vi "Parse Info Section.vi"(8 "error in":errorcluster, 11 "EDS in":refnum<class "EDS.lvclass">) -> (0 "error out":errorcluster, 3 "EDS out":refnum<class "EDS.lvclass">)   [LabVIEW 2024, in "EDS.lvlib" / "EDS.lvclass"]
uses:
  EDS.lvclass
  EDS.lvclass/EDS.ctl
  Device Info/Device Info.lvclass
  File Info/File Info.lvclass
  Info Section/Info Section.lvclass
  D:/git/EDS-File-Viewer/Core/Info Section/Info Section.lvclass
  D:/git/EDS-File-Viewer/Core/Device Info/Device Info.lvclass
  D:/git/EDS-File-Viewer/Core/File Info/File Info.lvclass
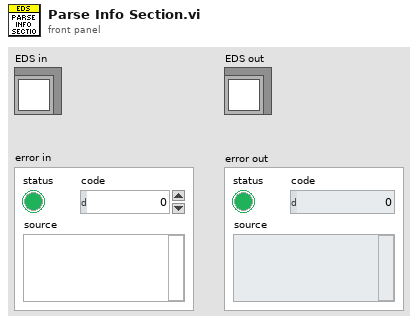
[diagram p1: front panel]
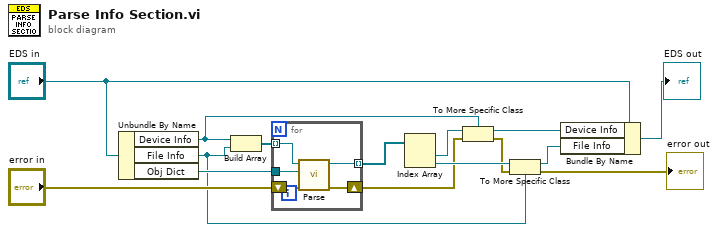
[diagram p0: block diagram]
diagram:
  n1 = Unbundle By Name("EDS in") -> ("Device Info"=w4:refnum<class "Device Info.lvclass">, "File Info"=w7:refnum<class "File Info.lvclass">, "Obj Dict"=w13:refnum<class "Object Dictionary.lvclass">)
  n2 = Build Array(w4, w7) -> (w8:refnum<class "Info Section.lvclass">[])
  n3 = for {
    tunnel: [w19] -> w14 mode=indexing
    tunnel: w13 -> [w18]
    shift-right: [w20] -> w2
    shift-left: "error in" -> [w17]
    tunnel: w8 -> [w16] mode=indexing
    n4 = call-dynamic "Parse.vi"("error in"=w17, "Object Dictionary"=w18, "Info Section in"=w16) -> ("error out"=w20:errorcluster, "Info Section out"=w19:refnum<class "Info Section.lvclass">)  [unwired: 7 in]
  }
  n5 = Index Array(array=w14) -> (element #1=w5:refnum<class "Info Section.lvclass">, element #2=w6:refnum<class "Info Section.lvclass">)  [unwired: 2 in]
  n6 = To More Specific Class(target class=w4, reference=w5, error in=w2) -> (specific class reference=w3:refnum<class "Device Info.lvclass">, error out=w1:errorcluster)
  n7 = To More Specific Class(target class=w7, reference=w6, error in=w1) -> (specific class reference=w11:refnum<class "File Info.lvclass">, error out=→"error out":errorcluster)
  n8 = Bundle By Name(cluster="EDS in", "Device Info"=w3, "File Info"=w11) -> (→"EDS out":refnum<class "EDS.lvclass">)
